vi "HDI Placement motion.vi"(7 "Console Log in":refnum<class "Console Log.lvclass">, 8 "error in":errorcluster, 11 "Gluing Procedure in":refnum<class "Gluing Procedure.lvclass">) -> (0 "error out":errorcluster, 1 "Step canceled?":bool, 3 "Gluing Procedure out":refnum<class "Gluing Procedure.lvclass">, 5 "Console Log out":refnum<class "Console Log.lvclass">)   [LabVIEW 2011, in "Gluing Procedure.lvclass"]
uses:
  Gluing Procedure.lvclass
  Application Utilities/Console Log/Console Log.lvclass
  Type Definitions/HDI Placement.ctl
  Shared Components/PickerTool Class/PickerTool Class.lvclass
panel:
  # "This VI does the HDI placement motion.\n\n1.  load picker\n2.  grab HDI\n3.  place HDI on BBM\n4.  return picker\n\nneed HDI -> BBM path motion (chuck/slot)"
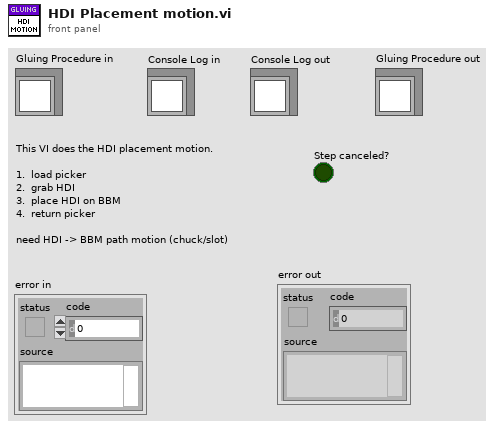
[diagram p1: front panel]
types:
  T1 = typedef "HDI Placement.ctl" = cluster{"Has been run?":bool}
  T2 = typedef "Configure.ctl" = cluster{"Has been run?":bool, "Active Paths":T3, "Glue Pathways":T4, "Chuck Module Used for BBM:":T6}
  T3 = typedef "Active Paths.ctl" = bool[]
  T4 = typedef "Glue Paths.ctl" = T5[]
  T5 = typedef "Glue Path.ctl" = cluster{"HDI Slot ":i32, "Stamp Slot":i32, "Glue Slot":i32, "Weight Slot":i32, "BBM Slot":i32}
  T6 = typedef "BBM Chuck Used.ctl" = i32
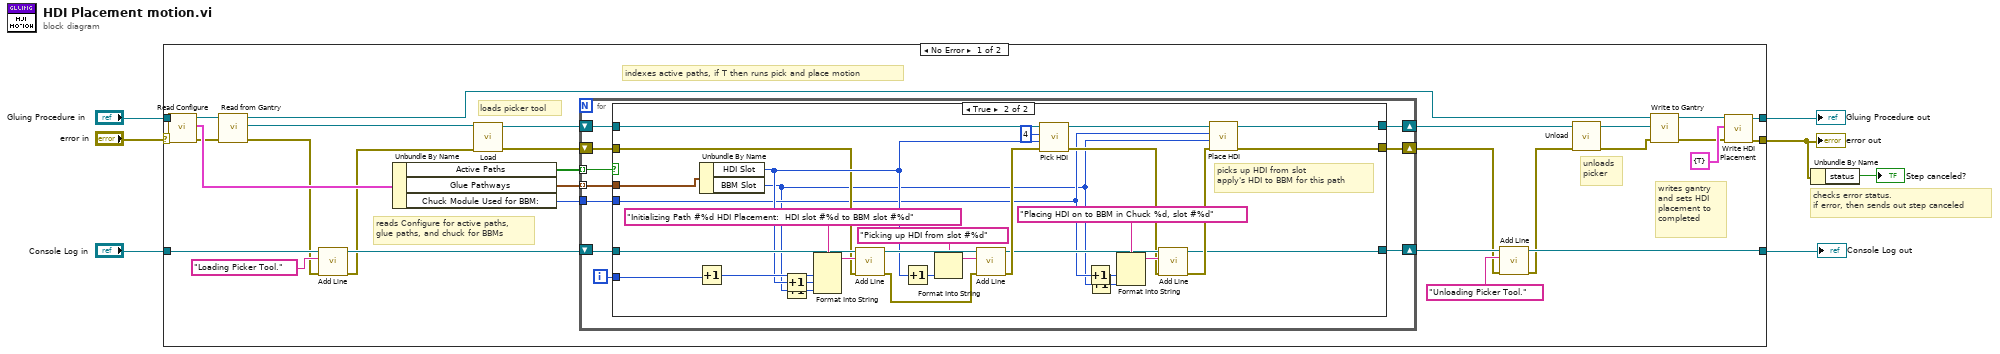
[diagram p0: block diagram]
diagram:
  # "checks error status.\nif error, then sends out step canceled"
  n1 = case shown="No Error" "error in" {
    selector: "error in" -> [w36 w84]
    tunnel: [w18 w84] -> w2
    tunnel: [w19 w83] -> w5
    tunnel: "Gluing Procedure in" -> [w37 w83]
    tunnel: [w11 w82] -> w4
    tunnel: "Console Log in" -> [w16 w82]
    frame No Error {
      # "indexes active paths, if T then runs pick and place motion"
      # "writes gantry\nand sets HDI\nplacement to \ncompleted"
      # "unloads\npicker"
      # "loads picker tool"
      # "reads Configure for active paths,\nglue paths, and chuck for BBMs"
      n2 = call "Read Configure.vi"("error in (no error)"=w36, "Gluing Procedure in"=w37) -> ("error out"=w32:errorcluster, "Configure"=w35:T2, "Gluing Procedure out"=w34:refnum<class "Gluing Procedure.lvclass">)  [unwired: 7 in]
      n3 = call "Read from Gantry.vi"("error in (no error)"=w32, "Gluing Procedure in"=w34) -> ("error out"=w14:errorcluster, "Gantry"=w33:refnum<class "Gantry Class.lvclass">, "Gluing Procedure out"=w24:refnum<class "Gluing Procedure.lvclass">)  [unwired: 7 in]
      n4 = call "Add Line.vi"("error in"=w14, "String"="Loading Picker Tool.", "Console Log in"=w16) -> ("error out"=w13:errorcluster, "Console Log out"=w15:refnum<class "Console Log.lvclass">)  [unwired: 7 in]
      n5 = Unbundle By Name(w35) -> ("Active Paths"=w29:T3, "Glue Pathways"=w28:T4, "Chuck Module Used for BBM:"=w27:T6)
      n6 = call "Load.vi"("error in"=w13, "Gantry in"=w33) -> ("error out"=w30:errorcluster, "PickerTool out"=w31:refnum<class "PickerTool Class.lvclass">)  [unwired: 8 in]
      n7 = for {
        shift-right: [w42] -> w26
        shift-left: w31 -> [w47]
        shift-right: [w41] -> w9
        shift-left: w30 -> [w46]
        tunnel: w29 -> [w45] mode=indexing
        tunnel: w28 -> [w44] mode=indexing
        tunnel: w27 -> [w43]
        shift-right: [w38] -> w12
        shift-left: w15 -> [w39]
        i -> [w40]
        n8 = case shown="True" w45 {
          tunnel: w47 -> [w50 w80]
          tunnel: w46 -> [w49 w64]
          tunnel: w44 -> [_ w81]
          tunnel: w43 -> [_ w55]
          tunnel: [w50 w77] -> w42
          tunnel: [w49 w76] -> w41
          tunnel: w40 -> [_ w75]
          tunnel: w39 -> [w48 w72]
          tunnel: [w48 w51] -> w38
          frame False {
          }
          frame True {
            # "picks up HDI from slot\napply's HDI to BBM for this path"
            n9 = Increment(x=w75) -> (x+1=w74:i32)
            n10 = Unbundle By Name(w81) -> ("HDI Slot"=w65:i32, "BBM Slot"=w53:i32)
            n11 = Increment(x=w65) -> (x+1=w68:i32)
            n12 = Increment(x=w53) -> (x+1=w67:i32)
            n13 = Format Into String(format string="Initializing Path #%d HDI Placement:  HDI slot #%d to BBM slot #%d", w74, w68, w67) -> (resulting string=w71:string)  [unwired: 2 in, 1 out]
            n14 = call "Add Line.vi"("error in"=w64, "String"=w71, "Console Log in"=w72) -> ("error out"=w63:errorcluster, "Console Log out"=w70:refnum<class "Console Log.lvclass">)  [unwired: 7 in]
            n15 = Increment(x=w65) -> (x+1=w66:i32)
            n16 = Format Into String(format string="Picking up HDI from slot #%d", w66) -> (resulting string=w69:string)  [unwired: 2 in, 1 out]
            n17 = call "Add Line.vi"("error in"=w63, "String"=w69, "Console Log in"=w70) -> ("error out"=w62:errorcluster, "Console Log out"=w57:refnum<class "Console Log.lvclass">)  [unwired: 7 in]
            n18 = call-dynamic "Pick HDI.vi"("error in"=w62, "Slot"=w65, "Chuck"=4, "PickerTool in"=w80) -> ("error out"=w56:errorcluster, "PickerTool out"=w78:refnum<class "PickerTool Class.lvclass">)  [unwired: 6 in]
            n19 = Increment(x=w55) -> (x+1=w59:T6)
            n20 = Increment(x=w53) -> (x+1=w54:i32)
            n21 = Format Into String(format string="Placing HDI on to BBM in Chuck %d, slot #%d", w59, w54) -> (resulting string=w58:string)  [unwired: 2 in, 1 out]
            n22 = call "Add Line.vi"("error in"=w56, "String"=w58, "Console Log in"=w57) -> ("error out"=w52:errorcluster, "Console Log out"=w51:refnum<class "Console Log.lvclass">)  [unwired: 7 in]
            n23 = call-dynamic "Place HDI.vi"("error in"=w52, "Slot Number"=w53, "Chuck Number"=w55, "PickupTool in"=w78) -> ("error out"=w76:errorcluster, "PickupTool out"=w77:refnum<class "PickerTool Class.lvclass">)  [unwired: 6 in]
          }
        }
      }
      n24 = call "Add Line.vi"("error in"=w9, "String"="Unloading Picker Tool.", "Console Log in"=w12) -> ("error out"=w8:errorcluster, "Console Log out"=w11:refnum<class "Console Log.lvclass">)  [unwired: 7 in]
      n25 = call "Unload.vi"("error in"=w8, "PickupTool in"=w26) -> ("error out"=w22:errorcluster, "Gantry out"=w25:refnum<class "Gantry Class.lvclass">)  [unwired: 8 in]
      n26 = call "Write to Gantry.vi"("error in (no error)"=w22, "Gantry"=w25, "Gluing Procedure in"=w24) -> ("error out"=w21:errorcluster, "Gluing Procedure out"=w20:refnum<class "Gluing Procedure.lvclass">)  [unwired: 7 in]
      n27 = call "Write HDI Placement.vi"("error in (no error)"=w21, "HDI Placement"=T1 {"Has been run?"=TRUE}, "Gluing Procedure in"=w20) -> ("error out"=w18:errorcluster, "Gluing Procedure out"=w19:refnum<class "Gluing Procedure.lvclass">)  [unwired: 7 in]
    }
    frame Error {
    }
  }
  "error out" <- w2
  "Gluing Procedure out" <- w5
  "Console Log out" <- w4
  n28 = Unbundle By Name(w2) -> ("status"=→"Step canceled?":bool)
